vi "from string.vi"(8 "error in":errorcluster, 9 "data":string, 10 "version":string, 11 "CVT Engine Configuration in":refnum<class "CVT Engine Configuration.lvclass">) -> (0 "error out":errorcluster, 3 "CVT Engine Configuration out":refnum<class "CVT Engine Configuration.lvclass">)   [LabVIEW 2013, in "CVT Engine Configuration.lvclass"]
doc: "Takes a version and data string and unflattens the data back into an Engine Configuration object."
uses:
  CVT Engine Configuration.lvclass
  <vilib>/NI/Module Execution Interface/Engine Configuration/engine configuration.lvclass
  <vilib>/NI/Configuration Framework/serializable configuration/NISE_CEF_serializable configuration.lvclass
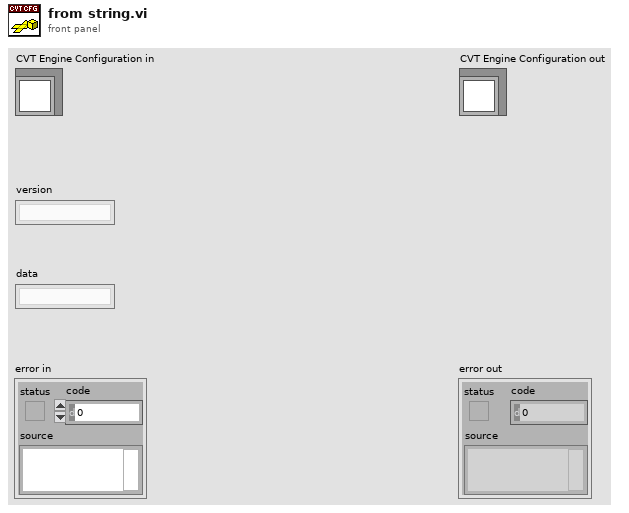
[diagram p1: front panel]
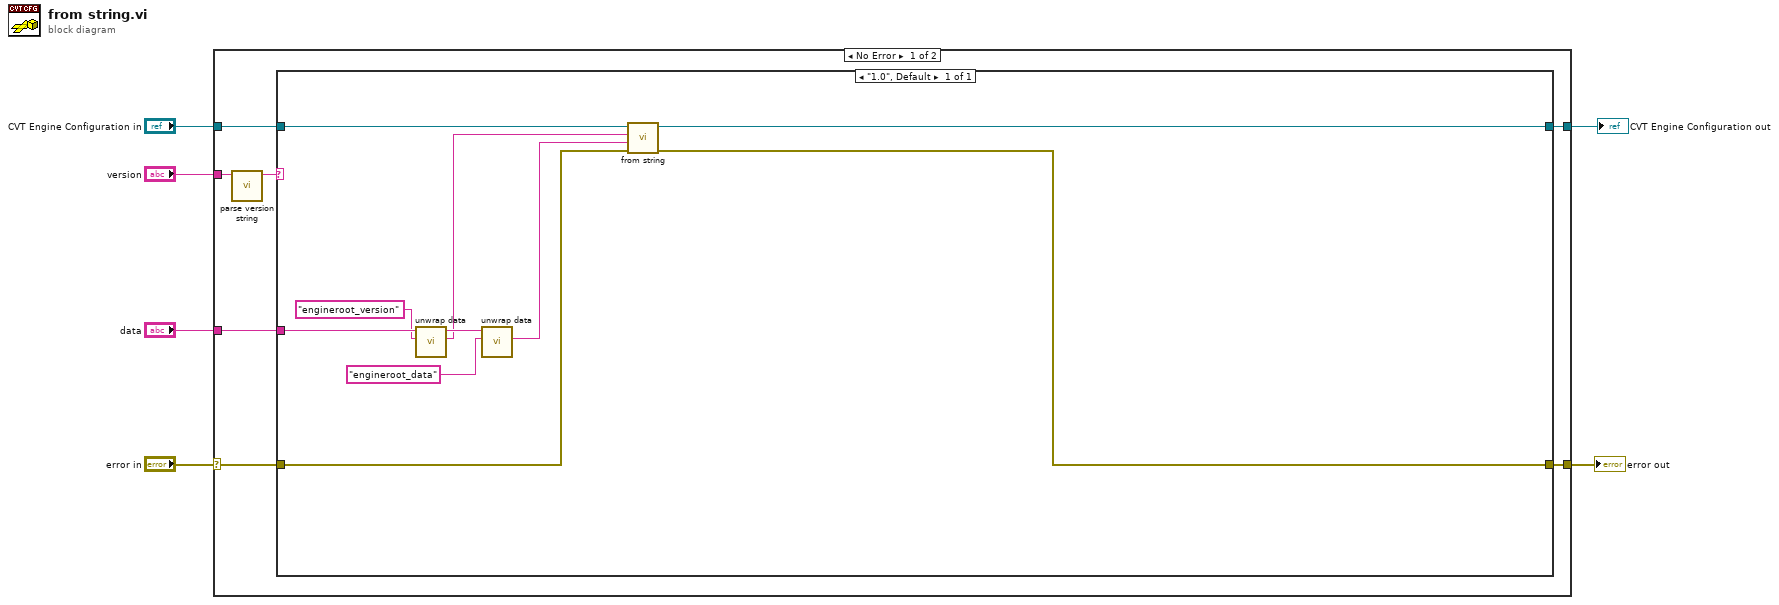
[diagram p0: block diagram]
diagram:
  n1 = case shown="No Error" "error in" {
    selector: "error in" -> [w7 w25]
    tunnel: "data" -> [w13 _]
    tunnel: "CVT Engine Configuration in" -> [w12 w24]
    tunnel: [w11 w24] -> w1
    tunnel: [w10 w25] -> w3
    tunnel: "version" -> [w9 _]
    frame No Error {
      n2 = call <vilib>:"parse version string.vi"("full version"=w9) -> ("major.minor version"=w8:string)  [unwired: 7 in, 3 out]
      n3 = case shown="\"1.0\", Default" w8 {
        tunnel: w7 -> [w23]
        tunnel: w13 -> [w20]
        tunnel: w12 -> [w22]
        tunnel: [w16] -> w11
        tunnel: [w17] -> w10
        frame "1.0", Default {
          n4 = call <vilib>:"unwrap data.vi"("identifier"="engineroot_version" ("additional identifier"), "data to unwrap"=w20) -> ("unwrapped data"=w19:string, "remaining string"=w21:string)  [unwired: 8 in]
          n5 = call <vilib>:"unwrap data.vi"("identifier"="engineroot_data" ("additional identifier"), "data to unwrap"=w21) -> ("unwrapped data"=w18:string)  [unwired: 8 in, 1 out]
          n6 = call-parent "from string.vi"("error in"=w23, "data"=w18, "version"=w19, "engine configuration in"=w22) -> ("error out"=w17:errorcluster, "engine configuration out"=w16:refnum<class "CVT Engine Configuration.lvclass">)  [unwired: 6 in]
        }
      }
    }
    frame Error {
    }
  }
  "error out" <- w3
  "CVT Engine Configuration out" <- w1
